vi "graphViz error dialog.vi"() -> ()   [LabVIEW 2013, in "PL Framework Configuration Tool.lvlib" / "Engine Mappings.lvclass"]
uses:
  Engine Mappings.lvclass
  <vilib>/Platform/browser.llb/Open URL in Default Browser (string).vi
panel:
  in  "OK Button":bool
  out "GraphViz Link":string="http://www.graphviz.org/Download_windows.php"
  out "Path Variable":string="Windows PATH variable"
  # "This visualization feature is not currently enabled. To enable this feature, install the open source GraphViz software from..."
  # "Once installed, register the Dot.exe with the"
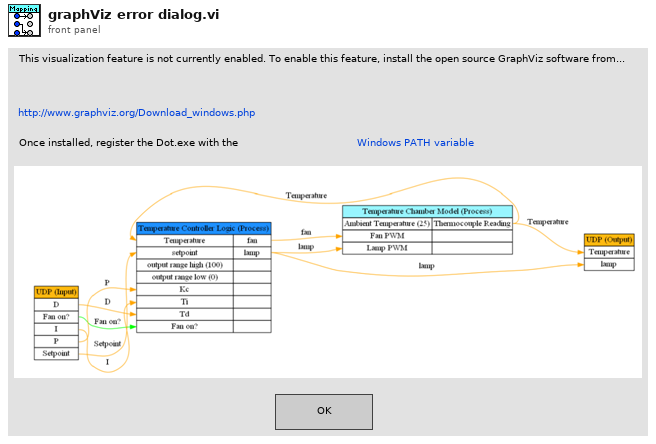
[diagram p1: front panel]
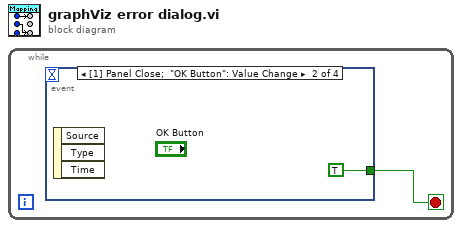
[diagram p0: block diagram]
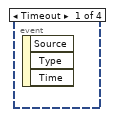
[diagram p2: hidden frame]
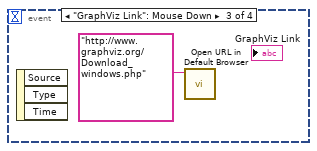
[diagram p3: hidden frame]
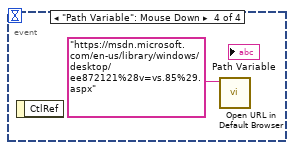
[diagram p4: hidden frame]
diagram:
  n1 = while {
    stop <- w1 stop-if-true
    n2 = event shown="[1] Panel Close;  \"OK Button\": Value Change" {
      selector: _ -> [_ _ _ _]
      dyn-events: _ -> [_ _ _ _]
      timeout: _ -> [_ _ _ _]
      tunnel: [_ TRUE _ _] -> w1
      event Timeout {
        n3 = event-data() -> ()  [unwired: 1 in, 3 out]
      }
      event Panel Close; "OK Button": Value Change {
        n4 = event-data() -> ()  [unwired: 1 in, 3 out]
      }
      event "GraphViz Link": Mouse Down {
        n5 = event-data() -> ()  [unwired: 1 in, 3 out]
        n6 = call-poly <vilib>:"Open URL in Default Browser.vi"("URL"="http://www.graphviz.org/Download_windows.php") -> ()  [unwired: 5 in, 2 out]
      }
      event "Path Variable": Mouse Down {
        n7 = event-data() -> ()  [unwired: 1 in, 1 out]
        n8 = call-poly <vilib>:"Open URL in Default Browser.vi"("URL"="https://msdn.microsoft.com/en-us/library/windows/desktop/ee872121%28v=vs.85%29.aspx") -> ()  [unwired: 5 in, 2 out]
      }
    }
  }
